vi "Zmienna FVG.vi"(7 "Akcja":enum16{"GET", "SET", "ADD"}(ring), 10 "Data in":dbl) -> (2 "Data out":dbl)   [LabVIEW 2013]
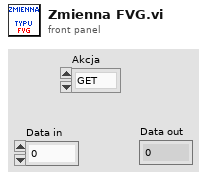
[diagram p1: front panel]
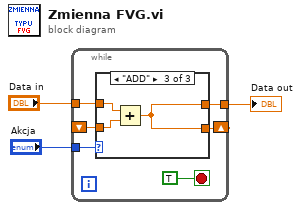
[diagram p0: block diagram]
diagram:
  n1 = while {
    tunnel: "Akcja" -> [w9]
    tunnel: "Data in" -> [w8]
    shift-right: [w7] -> _
    shift-left: _ -> [w6]
    tunnel: [w5] -> w1
    stop <- TRUE stop-if-true
    n2 = case shown="\"ADD\"" w9 {
      tunnel: w8 -> [_ w11 w14]
      tunnel: [w10 w11 w12] -> w7
      tunnel: w6 -> [w10 _ w13]
      tunnel: [w10 w11 w12] -> w5
      frame "GET", Default {
      }
      frame "SET" {
      }
      frame "ADD" {
        n3 = Add(x=w14, y=w13) -> (x+y=w12:dbl)
      }
    }
  }
  "Data out" <- w1
